vi "biref3.vi"() -> ()   [LabVIEW 2020]
uses:
  <vilib>/Utility/file.llb/Read From Spreadsheet File (DBL).vi
panel:
  out "dup directory path":path
  out "element":i32
  in  "Wait (second) to equilibrate temperature":sgl=100.0
  out "readfile":sgl[][](array[numeric]) format="%0.3f"
  in  "folder name":string="foldername"
  in  "field increment":dbl=1.0
  out "Current field":dbl
  in  "Initial field T":dbl=0.08
  in  "No  of field ramp Steps":i16=16
  out "outputdc 2":dbl[](array[numeric]) format="%.2f"
  in  "GPIB address dc meter 2":string="2"
  in  "GPIB address dc meter":string="5"
  in  "GPIB  address  lockin":string="3"
  in  "GPIB address magnet":string="1"
  in  "GPIB address Temp controller":string="12"
  in  "Wait (second) to ramp field up or down":sgl=10.0
  out "outputtemp":dbl[](array[numeric]) format="%.2f"
  out "outputdc":dbl[](array[numeric]) format="%.2f"
  out "outputlockin 2":dbl[](array[numeric]) format="%.2f"
  out "outputlockin 1":dbl[](array[numeric]) format="%.2f"
  out "field":dbl[](array[numeric]) format="%.2f"
  out "Current Temp":dbl format="%.3f"
  # "Help:\n1. write the folder name to save the files.The file name will \nbe the temperature in the given folder.\n2.Write the GPIB address of all the instruments before running\nthe program.\n3. Give the initial temperature and the temperature interval \nand the total number of steps.\n4.Check whether you want to increase the temperature or\ndecrease.\n5.Write the time to be waited to let the tempetature controller\nequilibrate.\n6.Once the speps 1 through 5 is done run the experiment."
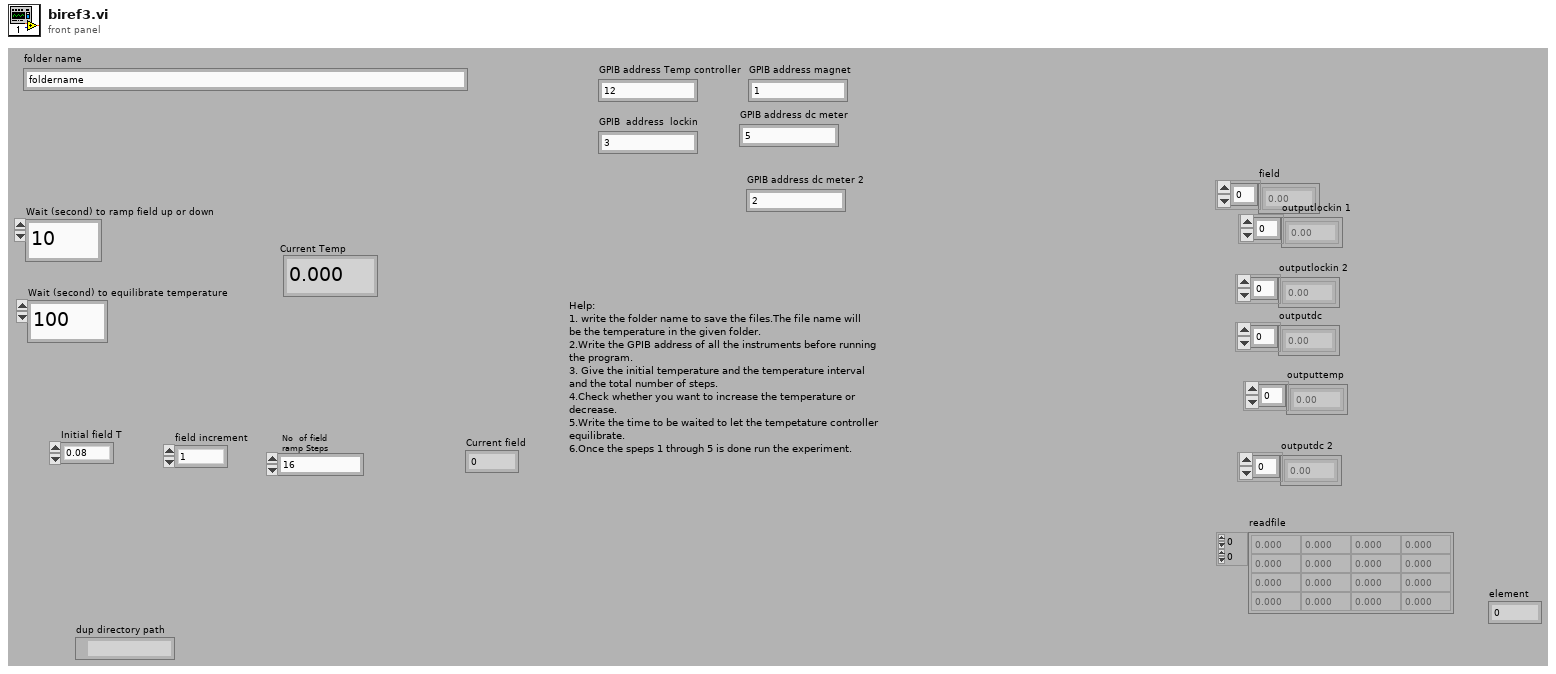
[diagram p1: front panel]
types:
  T1 = enum16{"--Quit--", "Read-Status", "Read-Cell", "Read-Field[T]", "Read-Setpoint[T]"}
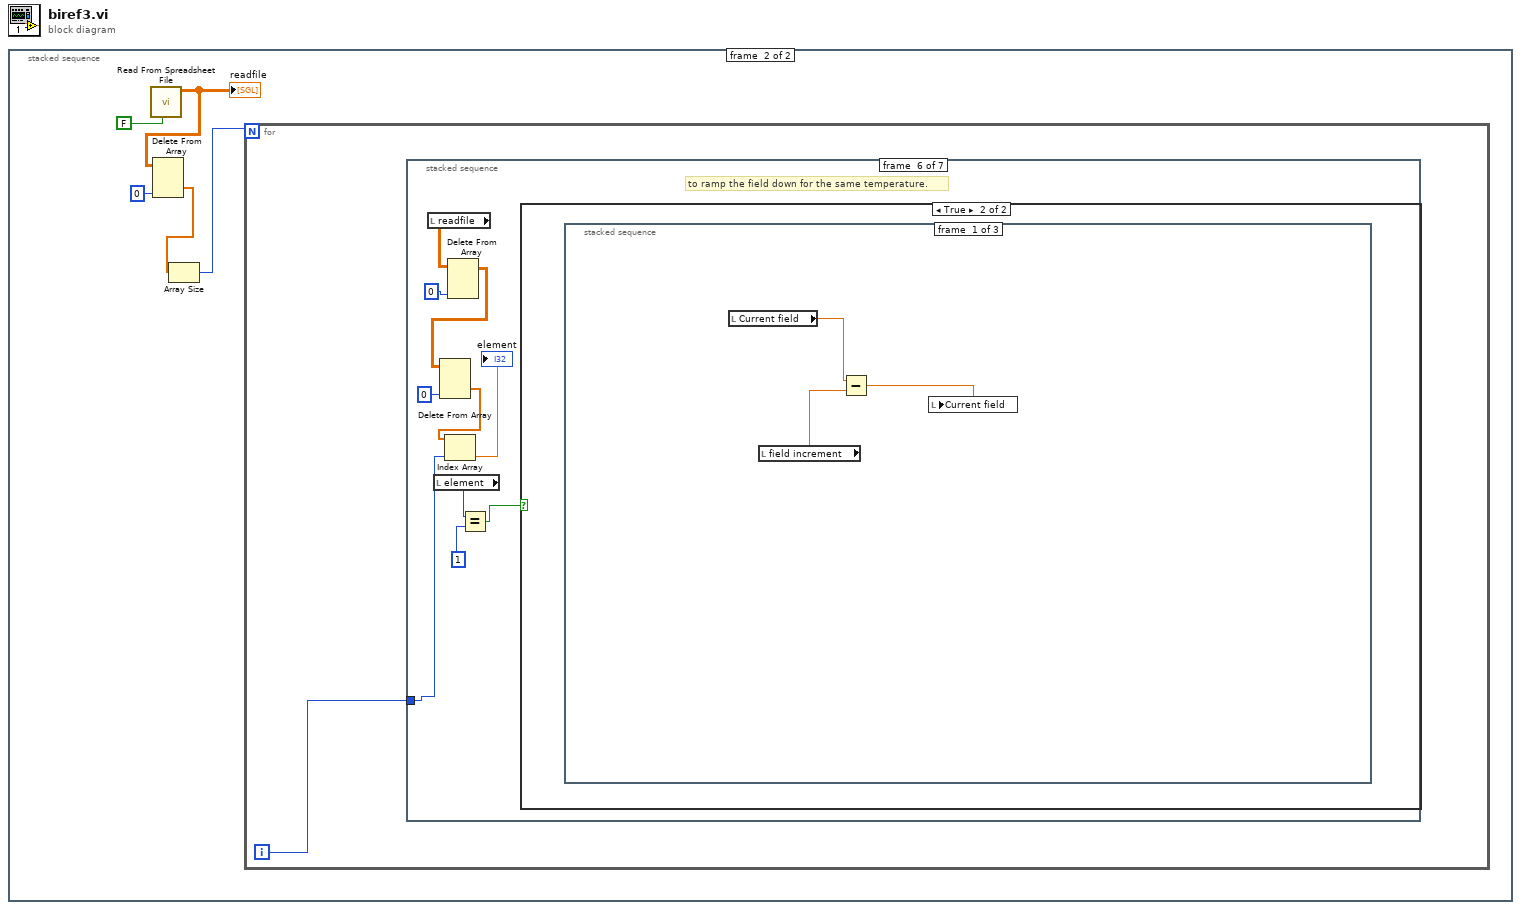
[diagram p0: block diagram]
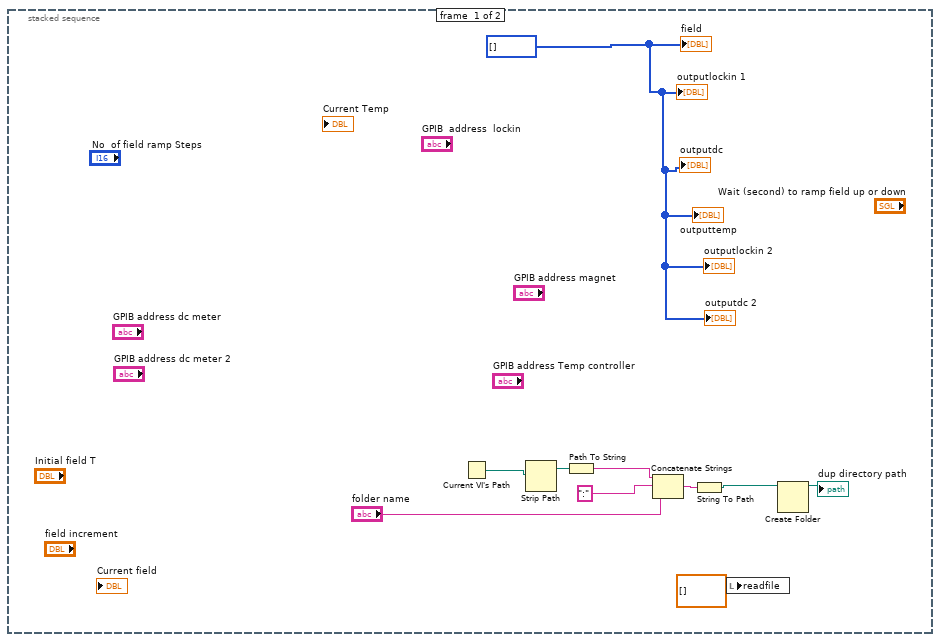
[diagram p2: hidden frame]
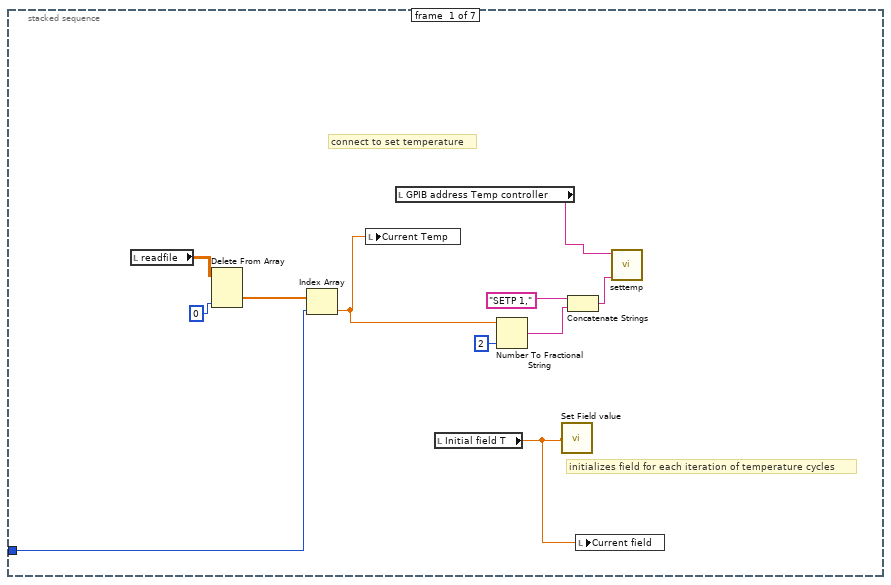
[diagram p3: hidden frame]
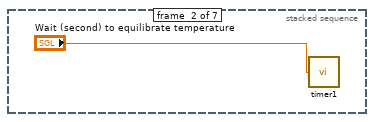
[diagram p4: hidden frame]
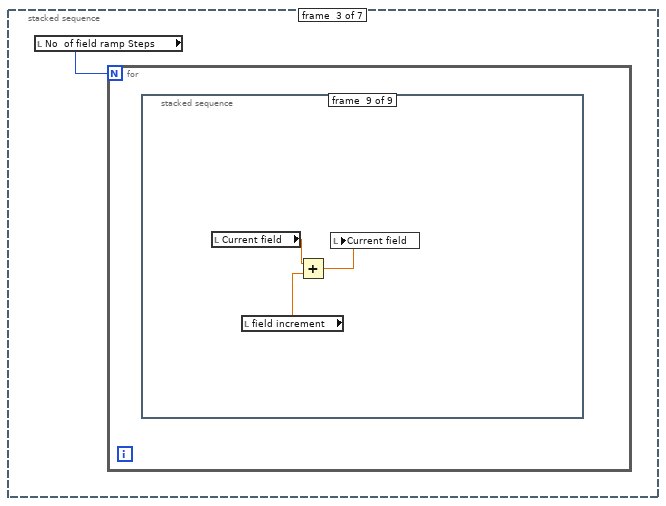
[diagram p5: hidden frame]
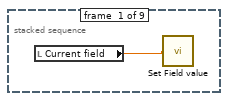
[diagram p6: hidden frame]
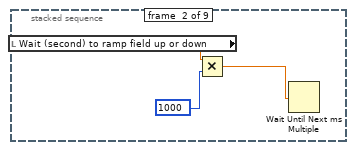
[diagram p7: hidden frame]
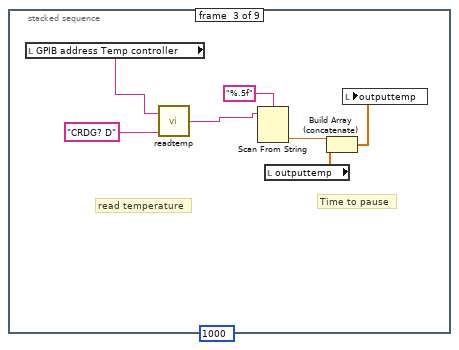
[diagram p8: hidden frame]
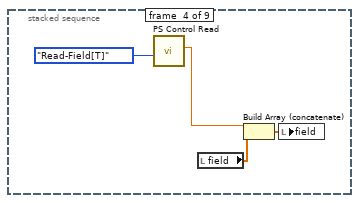
[diagram p9: hidden frame]
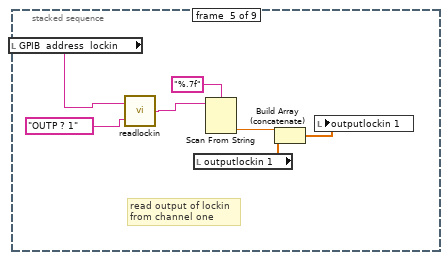
[diagram p10: hidden frame]
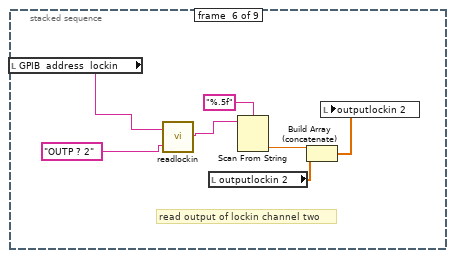
[diagram p11: hidden frame]
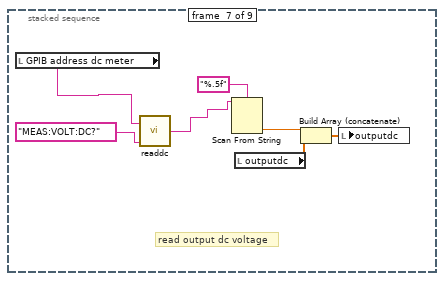
[diagram p12: hidden frame]
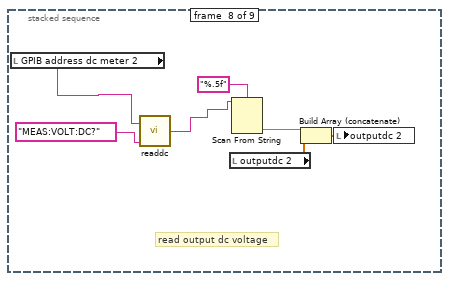
[diagram p13: hidden frame]
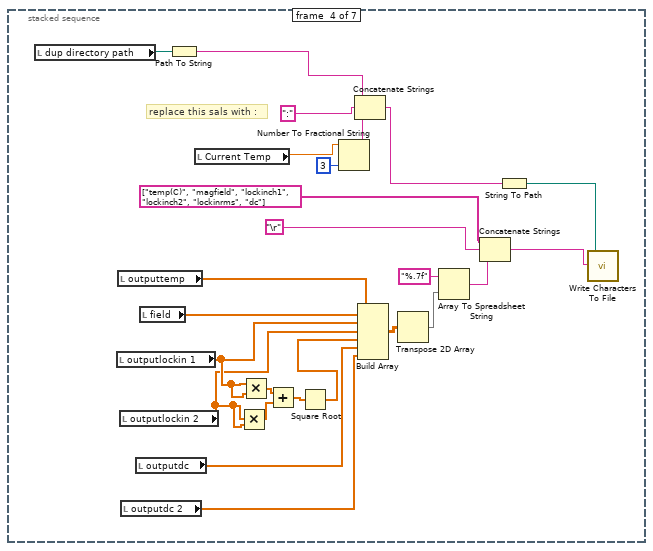
[diagram p14: hidden frame]
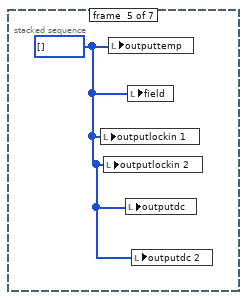
[diagram p15: hidden frame]
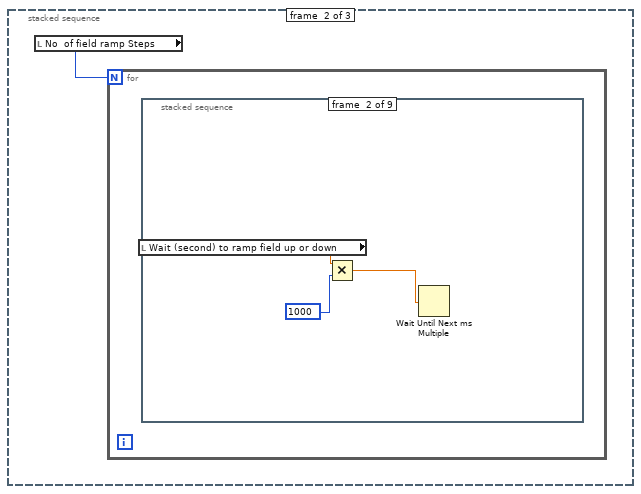
[diagram p17: hidden frame]
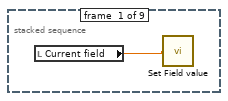
[diagram p18: hidden frame]
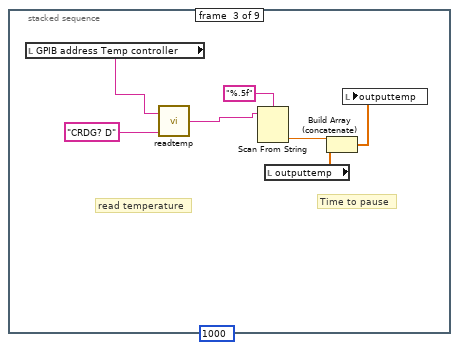
[diagram p19: hidden frame]
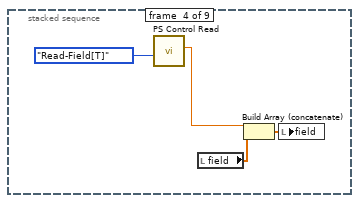
[diagram p20: hidden frame]
diagram:
  n1 = stacked-sequence {
    frame #0 {
      w10 = i32[] [] ("field")
      n2 = Current VI's Path() -> (path=w4:path)
      n3 = Strip Path(path=w4) -> (stripped path=w5:path)  [unwired: 1 out]
      n4 = Path To String(path=w5) -> (string=w6:string)
      n5 = Concatenate Strings(w6, ":", "folder name") -> (w8:string)
      n6 = String To Path(string=w8) -> (path=w2:path)
      n7 = local write "readfile"(sgl[][] [] ("readfile")) -> ()
      n8 = Create Folder(path (use dialog)=w2) -> (created path=→"dup directory path":path)  [unwired: 2 in, 2 out]
      "field" <- w10
      "outputlockin 1" <- w10
      "outputdc" <- w10
      "outputtemp" <- w10
      "outputlockin 2" <- w10
      "outputdc 2" <- w10
    }
    frame #1 {
      n9 = call-poly <vilib>:"Read From Spreadsheet File.vi"("transpose (no:F)"=FALSE) -> ("all rows"=w11:dbl[][])  [unwired: 6 in, 4 out]
      "readfile" <- w11
      n10 = Delete From Array(array=w11, index (col)=0 ("disabled index (col)")) -> (deleted portion=w13:dbl[])  [unwired: 2 in, 1 out]
      n11 = Array Size(array=w13) -> (size(s)=w12:i32)
      n12 = for {
        N: w12 -> [_]
        i -> [w16]
        n13 = stacked-sequence {
          tunnel: w16 -> [w25 _ _ _ _ w106 _]
          frame #0 {
            # "initializes field for each iteration of temperature cycles"
            # "connect to set temperature"
            n14 = local read "readfile"() -> (w26:sgl[][])
            n15 = Delete From Array(array=w26, index (col)=0 ("disabled index (col)")) -> (deleted portion=w24:sgl[])  [unwired: 2 in, 1 out]
            n16 = Index Array(array=w24, index=w25) -> (element=w20:sgl)
            n17 = local write "Current Temp"(w20) -> ()
            n18 = local read "GPIB address Temp controller"() -> (w21:string)
            n19 = local read "Initial field T"() -> (w17:dbl)
            n20 = Number To Fractional String(number=w20, precision (6)=i16 2) -> (F-format string=w18:string)  [unwired: 2 in]
            n21 = call "Set Field value.vi"("Field"=w17) -> ()
            n22 = Concatenate Strings("SETP 1,", w18) -> (w23:string)
            n23 = local write "Current field"(w17) -> ()
            n24 = call "settemp.vi"("Characters to Write"=w23, "GPIB\nAddress"=w21) -> ()  [unwired: 5 in, 1 out]
          }
          frame #1 {
            n25 = call "timer1.vi"("Numeric 2"="Wait (second) to equilibrate temperature") -> ()  [unwired: 1 in]
          }
          frame #2 {
            n26 = local read "No  of field ramp Steps"() -> (w29:i16)
            n27 = for {
              N: w29 -> [_]
              n28 = stacked-sequence {
                frame #0 {
                  n29 = local read "Current field"() -> (w30:dbl)
                  n30 = call "Set Field value.vi"("Field"=w30) -> ()
                }
                frame #1 {
                  n31 = local read "Wait (second) to ramp field up or down"() -> (w33:sgl)
                  n32 = Multiply(x=w33, y=u32 1000 ("millisecond multiple")) -> (x*y=w31:sgl)
                  n33 = Wait Until Next ms Multiple(millisecond multiple=w31) -> ()  [unwired: 1 out]
                }
                frame #2 {
                  (unwired) u32 1000 ("millisecond multiple")
                  # "Time to pause"
                  # "read temperature"
                  n34 = local read "GPIB address Temp controller"() -> (w34:string)
                  n35 = call "readtemp.vi"("Characters to Write"="CRDG? D", "GPIB\nAddress"=w34) -> ("Characters Read"=w35:string)
                  n36 = Scan From String(format string="%.5f", input string=w35) -> (output 1=w37:dbl)  [unwired: 3 in, 3 out]
                  n37 = local read "outputtemp"() -> (w40:dbl[])
                  n38 = Build Array (concatenate)(w37, w40) -> (w39:dbl[])
                  n39 = local write "outputtemp"(w39) -> ()
                }
                frame #3 {
                  n40 = call "PS Control Read.vi"("Read State"=T1."Read-Field[T]") -> ("Current Field"=w41:dbl)  [unwired: 3 in, 4 out]
                  n41 = local read "field"() -> (w43:dbl[])
                  n42 = Build Array (concatenate)(w41, w43) -> (w42:dbl[])
                  n43 = local write "field"(w42) -> ()
                }
                frame #4 {
                  # "read output of lockin\nfrom channel one"
                  n44 = local read "GPIB  address  lockin"() -> (w45:string)
                  n45 = call "readlockin.vi"("Characters to Write"="OUTP ? 1", "GPIB\nAddress"=w45) -> ("Characters Read"=w46:string)
                  n46 = local read "outputlockin 1"() -> (w50:dbl[])
                  n47 = Scan From String(format string="%.7f", input string=w46) -> (output 1=w47:dbl)  [unwired: 3 in, 3 out]
                  n48 = Build Array (concatenate)(w47, w50) -> (w49:dbl[])
                  n49 = local write "outputlockin 1"(w49) -> ()
                }
                frame #5 {
                  # "read output of lockin channel two"
                  n50 = local read "GPIB  address  lockin"() -> (w52:string)
                  n51 = call "readlockin.vi"("Characters to Write"="OUTP ? 2", "GPIB\nAddress"=w52) -> ("Characters Read"=w53:string)
                  n52 = local read "outputlockin 2"() -> (w57:dbl[])
                  n53 = Scan From String(format string="%.5f", input string=w53) -> (output 1=w55:dbl)  [unwired: 3 in, 3 out]
                  n54 = Build Array (concatenate)(w55, w57) -> (w56:dbl[])
                  n55 = local write "outputlockin 2"(w56) -> ()
                }
                frame #6 {
                  # "read output dc voltage"
                  n56 = local read "GPIB address dc meter"() -> (w59:string)
                  n57 = call "readdc.vi"("Characters to Write"="MEAS:VOLT:DC?", "GPIB\nAddress"=w59) -> ("Characters Read"=w60:string)
                  n58 = Scan From String(format string="%.5f", input string=w60) -> (output 1=w62:dbl)  [unwired: 3 in, 3 out]
                  n59 = local read "outputdc"() -> (w65:dbl[])
                  n60 = Build Array (concatenate)(w62, w65) -> (w64:dbl[])
                  n61 = local write "outputdc"(w64) -> ()
                }
                frame #7 {
                  # "read output dc voltage"
                  n62 = local read "GPIB address dc meter 2"() -> (w66:string)
                  n63 = call "readdc.vi"("Characters to Write"="MEAS:VOLT:DC?", "GPIB\nAddress"=w66) -> ("Characters Read"=w67:string)
                  n64 = local read "outputdc 2"() -> (w72:dbl[])
                  n65 = Scan From String(format string="%.5f", input string=w67) -> (output 1=w69:dbl)  [unwired: 3 in, 3 out]
                  n66 = Build Array (concatenate)(w69, w72) -> (w71:dbl[])
                  n67 = local write "outputdc 2"(w71) -> ()
                }
                frame #8 {
                  n68 = local read "Current field"() -> (w75:dbl)
                  n69 = local read "field increment"() -> (w74:dbl)
                  n70 = Add(x=w75, y=w74) -> (x+y=w73:dbl)
                  n71 = local write "Current field"(w73) -> ()
                }
              }
            }
          }
          frame #3 {
            # "replace this sals with :"
            n72 = local read "dup directory path"() -> (w77:path)
            n73 = local read "outputlockin 1"() -> (w93:dbl[])
            n74 = local read "outputtemp"() -> (w95:dbl[])
            n75 = local read "outputlockin 2"() -> (w92:dbl[])
            n76 = local read "outputdc 2"() -> (w78:dbl[])
            n77 = local read "outputdc"() -> (w87:dbl[])
            n78 = local read "field"() -> (w94:dbl[])
            n79 = Path To String(path=w77) -> (string=w76:string)
            n80 = local read "Current Temp"() -> (w97:dbl)
            n81 = Multiply(x=w92, y=w92) -> (x*y=w90:dbl[])
            n82 = Multiply(x=w93, y=w93) -> (x*y=w91:dbl[])
            n83 = Add(x=w91, y=w90) -> (x+y=w89:dbl[])
            n84 = Square Root(x=w89) -> (sqrt(x)=w88:dbl[])
            n85 = Number To Fractional String(number=w97, precision (6)=i16 3) -> (F-format string=w96:string)  [unwired: 2 in]
            n86 = Concatenate Strings(w76, ":", w96) -> (w99:string)
            n87 = Build Array(w95, w94, w93, w92, w88, w87, w78) -> (w86:dbl[][])
            n88 = Transpose 2D Array(2D array=w86) -> (transposed array=w84:dbl[][])
            n89 = Array To Spreadsheet String(array=w84, 3:"%.7f" ("format string")) -> (spreadsheet string=w81:string)  [unwired: 1 in]
            n90 = Concatenate Strings(string[] ["temp(C)", "magfield", "lockinch1", "lockinch2", "lockinrms", "dc"], "\r", w81) -> (w80:string)
            n91 = String To Path(string=w99) -> (path=w98:path)
            n92 = call <vilib>:"Write Characters To File.vi"("character string"=w80, "file path (dialog if empty)"=w98) -> ()  [unwired: 3 in, 1 out]
          }
          frame #4 {
            w101 = i32[] []
            n93 = local write "outputlockin 1"(w101) -> ()
            n94 = local write "outputlockin 2"(w101) -> ()
            n95 = local write "outputtemp"(w101) -> ()
            n96 = local write "outputdc"(w101) -> ()
            n97 = local write "field"(w101) -> ()
            n98 = local write "outputdc 2"(w101) -> ()
          }
          frame #5 {
            # "to ramp the field down for the same temperature."
            n99 = local read "readfile"() -> (w109:sgl[][])
            n100 = local read "element"() -> (w102:i32)
            n101 = Delete From Array(array=w109, index (col)=0 ("disabled index (col)")) -> (array with subset deleted=w108:sgl[][])  [unwired: 2 in, 1 out]
            n102 = Delete From Array(array=w108, index (col)=0 ("disabled index (col)")) -> (deleted portion=w107:sgl[])  [unwired: 2 in, 1 out]
            n103 = Index Array(array=w107, index=w106) -> (element=→"element":sgl)
            n104 = Equal?(x=w102, y=1) -> (x = y?=w104:bool)
            n105 = case shown="True" w104 {
              frame False {
              }
              frame True {
                n106 = stacked-sequence {
                  frame #0 {
                    n107 = local read "Current field"() -> (w114:dbl)
                    n108 = local read "field increment"() -> (w113:dbl)
                    n109 = Subtract(x=w114, y=w113) -> (x-y=w112:dbl)
                    n110 = local write "Current field"(w112) -> ()
                  }
                  frame #1 {
                    n111 = local read "No  of field ramp Steps"() -> (w115:i16)
                    n112 = for {
                      N: w115 -> [_]
                      n113 = stacked-sequence {
                        frame #0 {
                          n114 = local read "Current field"() -> (w116:dbl)
                          n115 = call "Set Field value.vi"("Field"=w116) -> ()
                        }
                        frame #1 {
                          n116 = local read "Wait (second) to ramp field up or down"() -> (w119:sgl)
                          n117 = Multiply(x=w119, y=u32 1000 ("millisecond multiple")) -> (x*y=w117:sgl)
                          n118 = Wait Until Next ms Multiple(millisecond multiple=w117) -> ()  [unwired: 1 out]
                        }
                        frame #2 {
                          (unwired) u32 1000 ("millisecond multiple")
                          # "Time to pause"
                          # "read temperature"
                          n119 = local read "GPIB address Temp controller"() -> (w120:string)
                          n120 = call "readtemp.vi"("Characters to Write"="CRDG? D", "GPIB\nAddress"=w120) -> ("Characters Read"=w121:string)
                          n121 = Scan From String(format string="%.5f", input string=w121) -> (output 1=w123:dbl)  [unwired: 3 in, 3 out]
                          n122 = local read "outputtemp"() -> (w126:dbl[])
                          n123 = Build Array (concatenate)(w123, w126) -> (w125:dbl[])
                          n124 = local write "outputtemp"(w125) -> ()
                        }
                        frame #3 {
                          n125 = call "PS Control Read.vi"("Read State"=T1."Read-Field[T]") -> ("Current Field"=w127:dbl)  [unwired: 3 in, 4 out]
                          n126 = local read "field"() -> (w129:dbl[])
                          n127 = Build Array (concatenate)(w127, w129) -> (w128:dbl[])
                          n128 = local write "field"(w128) -> ()
                        }
                        frame #4 {
                          # "read output of lockin\nfrom channel one"
                          n129 = local read "GPIB  address  lockin"() -> (w131:string)
                          n130 = call "readlockin.vi"("Characters to Write"="OUTP ? 1", "GPIB\nAddress"=w131) -> ("Characters Read"=w132:string)
                          n131 = local read "outputlockin 1"() -> (w136:dbl[])
                          n132 = Scan From String(format string="%.7f", input string=w132) -> (output 1=w133:dbl)  [unwired: 3 in, 3 out]
                          n133 = Build Array (concatenate)(w133, w136) -> (w135:dbl[])
                          n134 = local write "outputlockin 1"(w135) -> ()
                        }
                        frame #5 {
                          # "read output of lockin channel two"
                          n135 = local read "GPIB  address  lockin"() -> (w138:string)
                          n136 = call "readlockin.vi"("Characters to Write"="OUTP ? 2", "GPIB\nAddress"=w138) -> ("Characters Read"=w139:string)
                          n137 = local read "outputlockin 2"() -> (w143:dbl[])
                          n138 = Scan From String(format string="%.5f", input string=w139) -> (output 1=w141:dbl)  [unwired: 3 in, 3 out]
                          n139 = Build Array (concatenate)(w141, w143) -> (w142:dbl[])
                          n140 = local write "outputlockin 2"(w142) -> ()
                        }
                        frame #6 {
                          # "read output dc voltage"
                          n141 = local read "GPIB address dc meter"() -> (w145:string)
                          n142 = call "readdc.vi"("Characters to Write"="MEAS:VOLT:DC?", "GPIB\nAddress"=w145) -> ("Characters Read"=w146:string)
                          n143 = Scan From String(format string="%.5f", input string=w146) -> (output 1=w148:dbl)  [unwired: 3 in, 3 out]
                          n144 = local read "outputdc"() -> (w151:dbl[])
                          n145 = Build Array (concatenate)(w148, w151) -> (w150:dbl[])
                          n146 = local write "outputdc"(w150) -> ()
                        }
                        frame #7 {
                          # "read output dc voltage"
                          n147 = local read "GPIB address dc meter 2"() -> (w152:string)
                          n148 = call "readdc.vi"("Characters to Write"="MEAS:VOLT:DC?", "GPIB\nAddress"=w152) -> ("Characters Read"=w153:string)
                          n149 = local read "outputdc 2"() -> (w158:dbl[])
                          n150 = Scan From String(format string="%.5f", input string=w153) -> (output 1=w155:dbl)  [unwired: 3 in, 3 out]
                          n151 = Build Array (concatenate)(w155, w158) -> (w157:dbl[])
                          n152 = local write "outputdc 2"(w157) -> ()
                        }
                        frame #8 {
                          n153 = local read "Current field"() -> (w161:dbl)
                          n154 = local read "field increment"() -> (w160:dbl)
                          n155 = Subtract(x=w161, y=w160) -> (x-y=w159:dbl)
                          n156 = local write "Current field"(w159) -> ()
                        }
                      }
                    }
                  }
                  frame #2 {
                    # "replace this sals with :"
                    n157 = local read "dup directory path"() -> (w163:path)
                    n158 = Path To String(path=w163) -> (string=w162:string)
                    n159 = local read "outputlockin 1"() -> (w182:dbl[])
                    n160 = local read "outputtemp"() -> (w184:dbl[])
                    n161 = local read "outputlockin 2"() -> (w181:dbl[])
                    n162 = local read "outputdc 2"() -> (w167:dbl[])
                    n163 = local read "outputdc"() -> (w176:dbl[])
                    n164 = local read "field"() -> (w183:dbl[])
                    n165 = local read "Current Temp"() -> (w185:dbl)
                    n166 = Multiply(x=w181, y=w181) -> (x*y=w179:dbl[])
                    n167 = Multiply(x=w182, y=w182) -> (x*y=w180:dbl[])
                    n168 = Add(x=w180, y=w179) -> (x+y=w178:dbl[])
                    n169 = Square Root(x=w178) -> (sqrt(x)=w177:dbl[])
                    n170 = Number To Fractional String(number=w185, precision (6)=i16 3) -> (F-format string=w166:string)  [unwired: 2 in]
                    n171 = Concatenate Strings("fdn", w166) -> (w164:string)
                    n172 = Build Array(w184, w183, w182, w181, w177, w176, w167) -> (w175:dbl[][])
                    n173 = Concatenate Strings(w162, ":", w164) -> (w187:string)
                    n174 = Transpose 2D Array(2D array=w175) -> (transposed array=w173:dbl[][])
                    n175 = Array To Spreadsheet String(array=w173, 3:"%.7f" ("format string")) -> (spreadsheet string=w170:string)  [unwired: 1 in]
                    n176 = Concatenate Strings(string[] ["temp(C)", "magfield", "lockinch1", "lockinch2", "lockinrms", "dc"], "\r", w170) -> (w169:string)
                    n177 = String To Path(string=w187) -> (path=w186:path)
                    n178 = call <vilib>:"Write Characters To File.vi"("character string"=w169, "file path (dialog if empty)"=w186) -> ()  [unwired: 3 in, 1 out]
                  }
                }
              }
            }
          }
          frame #6 {
            w189 = i32[] []
            n179 = local write "outputlockin 1"(w189) -> ()
            n180 = local write "outputlockin 2"(w189) -> ()
            n181 = local write "outputtemp"(w189) -> ()
            n182 = local write "outputdc"(w189) -> ()
            n183 = local write "field"(w189) -> ()
            n184 = local write "outputdc 2"(w189) -> ()
          }
        }
      }
    }
  }
